vi "Initialize DAQMan.vi"(8 "error in (no error)":errorcluster, 11 "Cfg Grandmaster in":refnum<class "Cfg Grandmaster.lvclass">) -> (0 "error out":errorcluster, 3 "Cfg Grandmaster out":refnum<class "Cfg Grandmaster.lvclass">)   [LabVIEW 2018, in "Configuration Grandmaster.lvlib" / "Cfg Grandmaster.lvclass"]
uses:
  Cfg Grandmaster.lvclass
  Cfg Grandmaster.lvclass/Cfg Grandmaster.ctl
  Common/Controls/DAQMan Mode.ctl
  TCP Server/TCP Connection Messages/Update Meta data Msg/Update Meta data Msg.lvclass/Update Meta data Msg.ctl
  <vilib>/ActorFramework/Message Enqueuer/Message Enqueuer.lvclass/Message Enqueuer.ctl
  <vilib>/ActorFramework/Message Enqueuer/Enqueue.vi
  TCP Server/TCP Connection Messages/Update Meta data Msg/Update Meta data Msg.lvclass
  C:/Program Files (x86)/National Instruments/LabVIEW 2018/vi.lib/ActorFramework/Message/Message.lvclass
  <vilib>/ActorFramework/Message Priority Queue/Priority Enqueue.vi
  Class FP Ctrls/FP Controls.lvclass
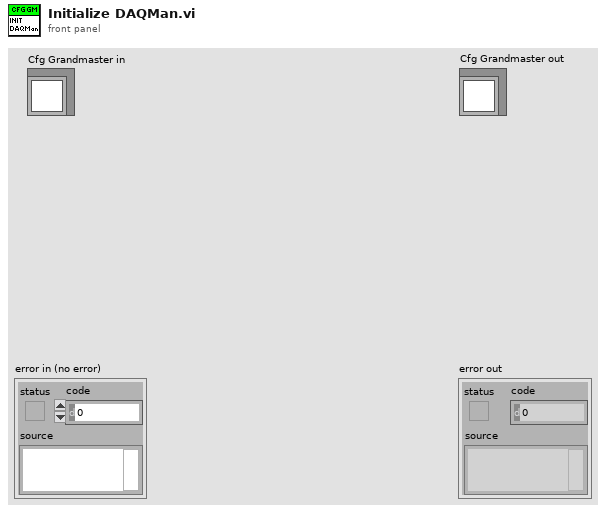
[diagram p1: front panel]
types:
  T1 = typedef "DAQMan Mode.ctl" = enum16{"Cfg", "Run", "Shutting Down"}
  T2 = typedef "ge_Cfg wChassis.ctl" = cluster{"Chassis BOM":refnum<class "Chassis BOM.lvclass">, "Chassis Cfg":refnum<class "ChassisCfg.lvclass">, "Chassis Tasks":refnum<class "Chassis Tasks.lvclass">, "HW Error":bool, "Unsvd Chgs?":bool}
  T3 = typedef "stm_MetaDataElement.ctl" = string
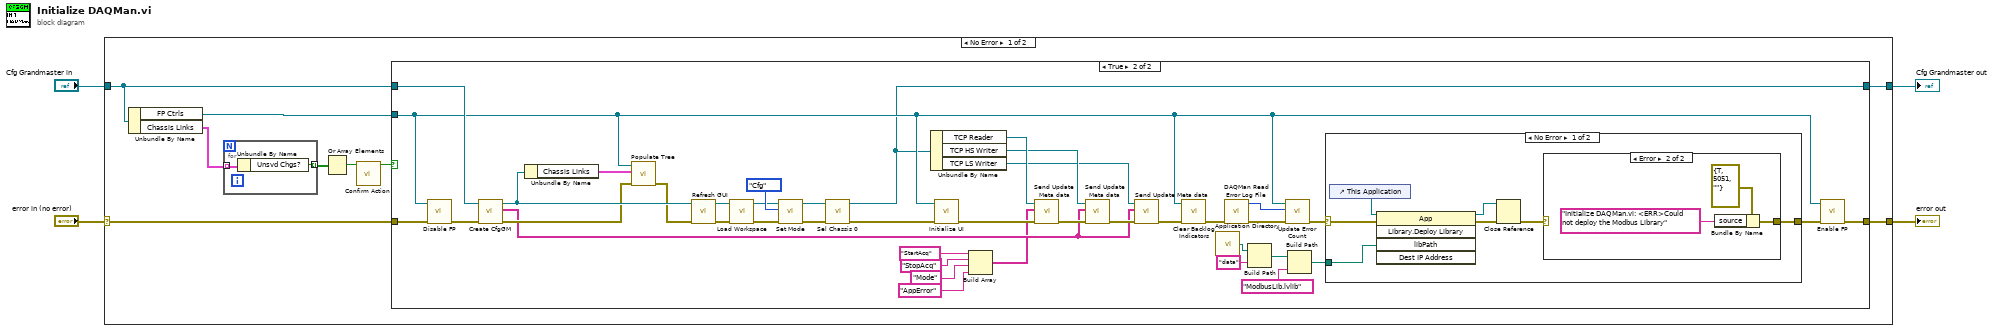
[diagram p0: block diagram]
diagram:
  n1 = case shown="No Error" "error in (no error)" {
    selector: "error in (no error)" -> [w13 w72]
    tunnel: [w12 w72] -> w3
    tunnel: [w10 w71] -> w1
    tunnel: "Cfg Grandmaster in" -> [w9 w71]
    frame No Error {
      n2 = Unbundle By Name(w9) -> ("FP Ctrls"=w11:refnum<class "FP Controls.lvclass">, "Chassis Links"=w7:T2[])
      n3 = for {
        tunnel: w7 -> [w70] mode=indexing
        tunnel: [w69] -> w8 mode=indexing
        n4 = Unbundle By Name(w70) -> ("Unsvd Chgs?"=w69:bool)
      }
      n5 = Or Array Elements(Boolean array=w8) -> (logical OR=w6:bool)
      n6 = call "Confirm Action.vi"("Confirm?"=w6) -> ("T button?"=w5:bool)  [unwired: 10 in]
      n7 = case shown="True" w5 {
        tunnel: w13 -> [w15 w46]
        tunnel: [w15 w43] -> w12
        tunnel: w11 -> [_ w29]
        tunnel: [w14 w17] -> w10
        tunnel: w9 -> [w14 w47]
        frame False {
        }
        frame True {
          n8 = call "Disable FP.vi"("error in (no error)"=w46, "FP Controls in"=w29) -> ("error out"=w45:errorcluster)  [unwired: 8 in, 1 out]
          n9 = call "Create CfgGM.vi"("error in (no error)"=w45, "Cfg Grandmaster in"=w47) -> ("error out"=w40:errorcluster, "Writer Meta data"=w32:T3[], "Cfg Grandmaster out"=w41:refnum<class "Cfg Grandmaster.lvclass">)  [unwired: 7 in]
          n10 = Unbundle By Name(w41) -> ("Chassis Links"=w42:T2[])
          n11 = call "Populate Tree.vi"("error in"=w40, "cDAQ Configs"=w42, "FP Controls"=w29) -> ("error out"=w39:errorcluster)  [unwired: 7 in, 1 out]
          n12 = call "Refresh GUI.vi"("error in (no error)"=w39, "Cfg Grandmaster in"=w41) -> ("error out"=w49:errorcluster, "Cfg Grandmaster out"=w48:refnum<class "Cfg Grandmaster.lvclass">)  [unwired: 8 in]
          n13 = call "Load Workspace.vi"("error in (no error)"=w49, "Cfg Grandmaster in"=w48) -> ("error out"=w20:errorcluster, "Cfg Grandmaster out"=w21:refnum<class "Cfg Grandmaster.lvclass">)  [unwired: 8 in]
          n14 = call "Set Mode.vi"("error in (no error)"=w20, "Mode"=DAQMan_Mode."Cfg", "Cfg Grandmaster in"=w21) -> ("error out"=w18:errorcluster, "Cfg Grandmaster out"=w19:refnum<class "Cfg Grandmaster.lvclass">)  [unwired: 7 in]
          n15 = call "Sel Chassis 0.vi"("error in (no error)"=w18, "Cfg Grandmaster in"=w19) -> ("error out"=w16:errorcluster, "Cfg Grandmaster out"=w17:refnum<class "Cfg Grandmaster.lvclass">)  [unwired: 8 in]
          n16 = Unbundle By Name(w17) -> ("TCP Reader"=w35:refnum<class "Message Enqueuer.lvclass">, "TCP HS Writer"=w34:refnum<class "Message Enqueuer.lvclass">, "TCP LS Writer"=w33:refnum<class "Message Enqueuer.lvclass">)
          n17 = call "Initialize UI.vi"("error in (no error)"=w16, "FP Controls in"=w29) -> ("error out"=w38:errorcluster)  [unwired: 8 in, 1 out]
          n18 = Build Array("StartAcq", "StopAcq", "Mode", "AppError") -> (w31:string[])
          n19 = call "Send Update Meta data.vi"("error in (no error)"=w38, "Meta data"=w31, "Message Enqueuer"=w35) -> ("error out"=w37:errorcluster)  [unwired: 7 in, 1 out]
          n20 = call "Send Update Meta data.vi"("error in (no error)"=w37, "Meta data"=w32, "Message Enqueuer"=w34) -> ("error out"=w36:errorcluster)  [unwired: 7 in, 1 out]
          n21 = call "Send Update Meta data.vi"("error in (no error)"=w36, "Meta data"=w32, "Message Enqueuer"=w33) -> ("error out"=w30:errorcluster)  [unwired: 7 in, 1 out]
          n22 = call "Clear Backlog Indicators.vi"("error in (no error)"=w30, "FP Controls in"=w29) -> ("error out"=w28:errorcluster)  [unwired: 8 in, 1 out]
          n23 = call <vilib>:"Application Directory.vi"() -> ("Application Directory"=w50:path)
          n24 = call "DAQMan Read Error Log File.vi"("error in (no error)"=w28) -> ("error out"=w27:errorcluster, "Number of Rows"=w26:u32)  [unwired: 8 in, 1 out]
          n25 = Build Path(base path=w50, name or relative path="data") -> (appended path=w52:path)
          n26 = call "Update Error Count.vi"("error in (no error)"=w27, "Error Count"=w26, "FP Controls in"=w29) -> ("error out"=w23:errorcluster)  [unwired: 7 in, 1 out]
          n27 = Build Path(base path=w52, name or relative path="ModbusLib.lvlib") -> (appended path=w54:path)
          n28 = case shown="No Error" w23 {
            selector: w23 -> [w60 w68]
            tunnel: w54 -> [w61 _]
            tunnel: [w58 w68] -> w44
            frame No Error {
              n29 = control-ref of="This Application"() -> (w57:refnum<vi>)
              n30 = invoke class="App" method="Library.Deploy Library"(reference=w57, error in=w60, "libPath"=w61) -> (reference out=w63:refnum<vi>, error out=w62:errorcluster)  [unwired: 2 in, 3 out]
              n31 = Close Reference(reference=w63, error in (no error)=w62) -> (error out=w59:errorcluster)
              n32 = case shown="Error" w59 {
                selector: w59 -> [w64 _]
                tunnel: [w64 w66] -> w58
                frame No Error {
                }
                frame Error {
                  n33 = Bundle By Name(cluster=errorcluster {"status"=TRUE, "code"=5051, "source"=""} ("error IO"), "source"="Initialize DAQMan.vi: <ERR>Could not deploy the Modbus Library") -> (w66:errorcluster)
                }
              }
            }
            frame Error {
            }
          }
          n34 = call "Enable FP.vi"("error in (no error)"=w44, "FP Controls in"=w29) -> ("error out"=w43:errorcluster)  [unwired: 8 in, 1 out]
        }
      }
    }
    frame Error {
    }
  }
  "error out" <- w3
  "Cfg Grandmaster out" <- w1
